vi "Main_PXI_Test.vi"() -> ()   [LabVIEW 2018]
doc: "Main VI for the controls"
uses:
  components/PMCL Dynamic Signal Analyzer/Controls/DSA excitation specs.ctl
  components/PMCL Dynamic Signal Analyzer/Controls/DSA cycle specs.ctl
  Typedefs/StateDef_Enum.ctl
  <vilib>/Utility/error.llb/DialogType.ctl
  <vilib>/Platform/TimedLoop/XDataNode/timing_clust.ctl
  <vilib>/Platform/TimedLoop/XDataNode/nitl_modes.ctl
  <vilib>/Platform/TimedLoop/XDataNode/wakeup.ctl
  <vilib>/DAQmx/read.llb/DAQmx Read (Analog 1D DBL NChan 1Samp).vi
  <vilib>/DAQmx/write.llb/DAQmx Write (Analog DBL 1Chan 1Samp).vi
  <vilib>/DAQmx/create/channels.llb/DAQmx Create Channel (AO-Voltage-Basic).vi
  <vilib>/DAQmx/create/channels.llb/DAQmx Create Channel (AI-Voltage-Basic).vi
  <vilib>/DAQmx/configure/timing.llb/DAQmx Timing (Sample Clock).vi
  <vilib>/DAQmx/create/timing.llb/DAQmx Create Timing Source (Control Loop From Task).vi
  <vilib>/DAQmx/miscellaneous.llb/DAQmx Fill In Error Info.vi
  <vilib>/Platform/TimedLoop/XDataNode/XDataNode.xnode
  Components/Timing/Timing.lvlib
  <vilib>/Platform/TimedLoop/XDataNode/XDNodeRunTimeDep.lvlib
  <vilib>/Analysis/NI_AALPro.lvlib
  <vilib>/ptbypt/NI_PtbyPt.lvlib
  <resource>/objmgr/daqmx.rc
panel:
  in  "System Stop Button":bool
  in  "Pause chart?":bool
  in  "Controller Params":enum32{"Page 1"}(tab)
  in  "Kp":dbl=1.0 min=0.0
  in  "Controller On?":bool
  out "Status":string
  in  "Ref. Gen.":enum32{"Analog In", "Manual", "Wave Gen", "DSA"}(tab)=enum."Manual"
  in  "Ref. cmd.":dbl(slide) step=1.0 scale=-10.0..10.0 scale format="%#.1f"
  in  "Signal Cluster":T1={"phase"=0.0, "amplitude"=1.0, "frequency"=1.0, "offset"=1.0, "Signal"=enum."Square"} {"offset" format="%0.2f"; "frequency" format="%0.2f"; "amplitude" format="%0.2f"; "phase" format="%0.2f"}
  in  "Frequency\nResponse":enum16{"Plant", "RR", "CL"}(ring)
  out "DSA \nRunning?":bool
  in  "Stop \nDSA":bool
  in  "Start \nDSA":bool
  in  "DSA excitation specs":T2={"Initial Freq. [Hz]"=10.0, "Final Freq. [Hz]"=999.0, "# pts. in interval"=50, "Samping Time [s]"=0.001, "Amplitude [V]"=1.0, "Offset [V]"=0.0, "Freq Units (F: rad/s, T: Hz)"=TRUE}
  in  "Cycle Specs":T3={"Cycles To \nSettle (M)"=5, "Cycles To \nCalculate (N)"=10}
  in  "Loop Timing":enum32{"Ctrl.", "Ref. gen", "UI"}(tab)
  in  "Ctrl.\nLoop Rate (Hz)":dbl=25000.0 format="%#_4p"
  out "# Finished\nLate counter":dbl
  in  "ConvLateErrToWarning?":bool=TRUE
  out "# Finished\nLate counter":dbl
  in  "Ref. Gen.\nLoop Rate (Hz)":dbl=20000.0 format="%#_4p"
  in  "UI Loop rate (Hz)":dbl=1000.0 format="%#_6p"
  in  "Display Waveforms":enum32{"Controller Signals", "DSA "}(tab)
  out "Control Effort":dbl(graph)
  out "Waveform Chart":cluster{"Double":dbl, "Numeric":dbl}(graph)
  out "Phase Bode Plot":cluster{dbl[], dbl[]}(graph)
  out "Magnitude Bode Plot":cluster{dbl[], dbl[]}(graph)
  out "DSA Signals":cluster{"Double":dbl, "Double":dbl}(graph)
  # "Connect the Reference Signal \nto C/AI 1 of the myRIO."
  # "Pinout Config.:\nPort C/AI0 : Plant output being read           by the controller.\nPort C/AI1 : Reference signal for the control loop.\nPort C/AO0 : Control effort signal to the plant."
  # "Control Loop Timing"
  # "Ref.  Gen. Loop Timing"
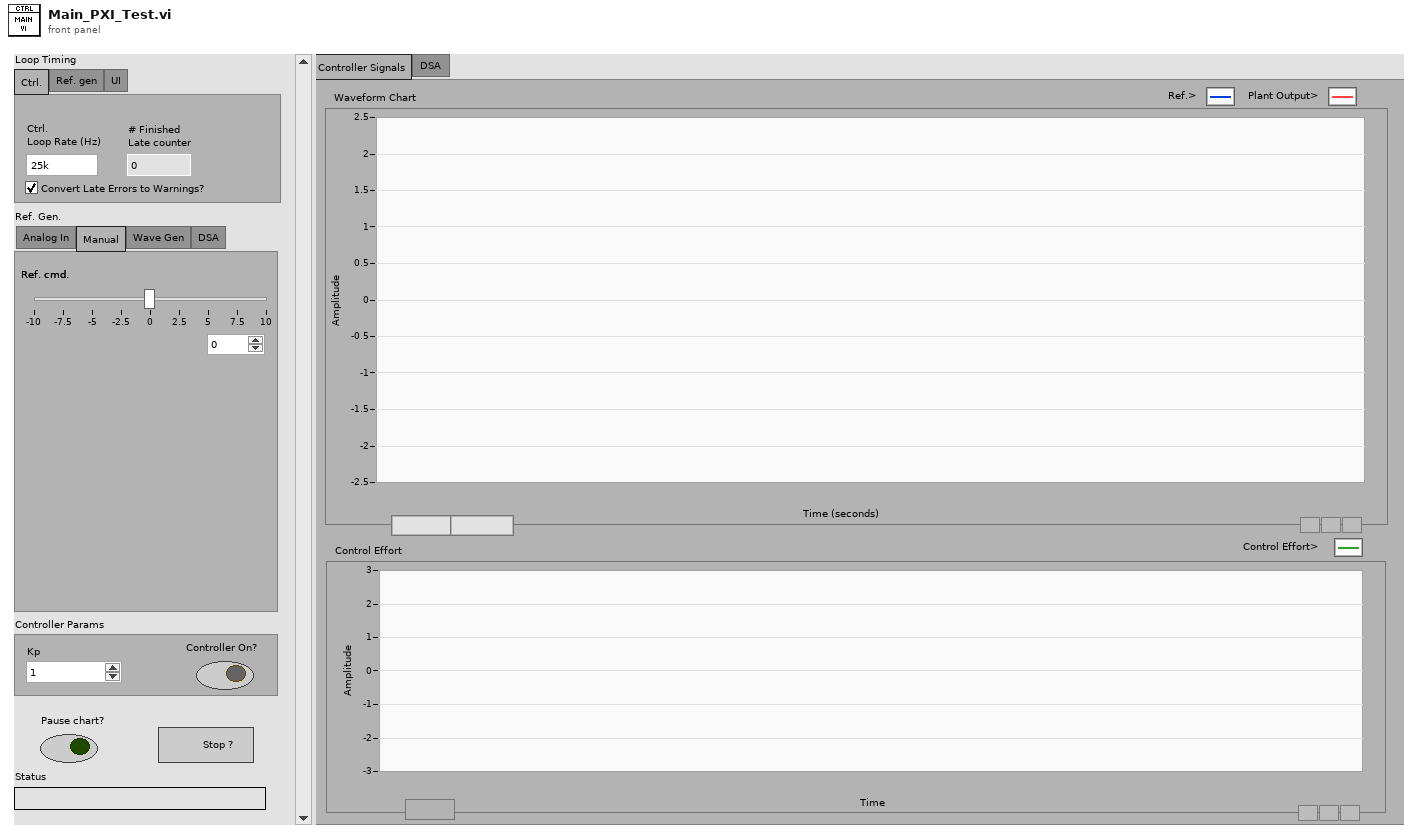
[diagram p1: front panel]
types:
  T1 = cluster{"phase":dbl, "amplitude":dbl, "frequency":dbl, "offset":dbl, "Signal":enum16{"Sine", "Square", "Sawtooth"}}
  T2 = typedef "DSA excitation specs.ctl" = cluster{"Initial Freq. [Hz]":dbl, "Final Freq. [Hz]":dbl, "# pts. in interval":i16, "Samping Time [s]":dbl, "Amplitude [V]":dbl, "Offset [V]":dbl, "Freq Units (F: rad/s, T: Hz)":bool}
  T3 = typedef "DSA cycle specs.ctl" = cluster{"Cycles To \nSettle (M)":i16, "Cycles To \nCalculate (N)":i16}
  T4 = typedef "DialogType.ctl" = u16
  T5 = typedef "StateDef_Enum.ctl" = enum16{"Initialize", "Wait", "Shutdown"}
  T6 = typedef "XDNodeRunTimeDep.lvlib/timing_clust.ctl" = cluster{"Expected End [f-1]":u64, "Actual End [f-1]":u64, "Finished Late? [f-1]":bool, "Expected End [i-1]":u64, "Actual End [i-1]":u64, "Finished Late? [i-1]":bool, "Expected Start [i]":u64, "Actual Start [i]":u64, "Expected Start [f]":u64, "Actual Start [f]":u64, "Source Name":string, "Structure Name":string, "Period":i64, "Deadline":i64, "Offset":i64, "Start":i64, "Priority":i32, "Timeout":i32, "Mode":T7, "Wakeup Reason":T8, "Error":errorcluster, "Source Type":string, "Secondary Source Type":string, "Global End Time":u64, "Global Start Time":u64, "Frame Duration":u64, "Iteration Duration":u64, "Assigned CPU":i32, "I/O Scan Engine Mode":u32}
  T7 = typedef "XDNodeRunTimeDep.lvlib/nitl_modes.ctl" = enum32{"No Change", "Process missed periods, maintain original phase", "Discard missed periods, maintain original phase", "Process missed periods, ignore original phase", "Discard missed periods, ignore original phase"}
  T8 = typedef "XDNodeRunTimeDep.lvlib/wakeup.ctl" = enum32{"Normal", "Aborted", "Asynchronous wakeup", "Timing source error", "Timed loop error", "Timeout"}
  T9 = cluster{"Analog In CH1":dbl, "Analog In CH0":dbl}
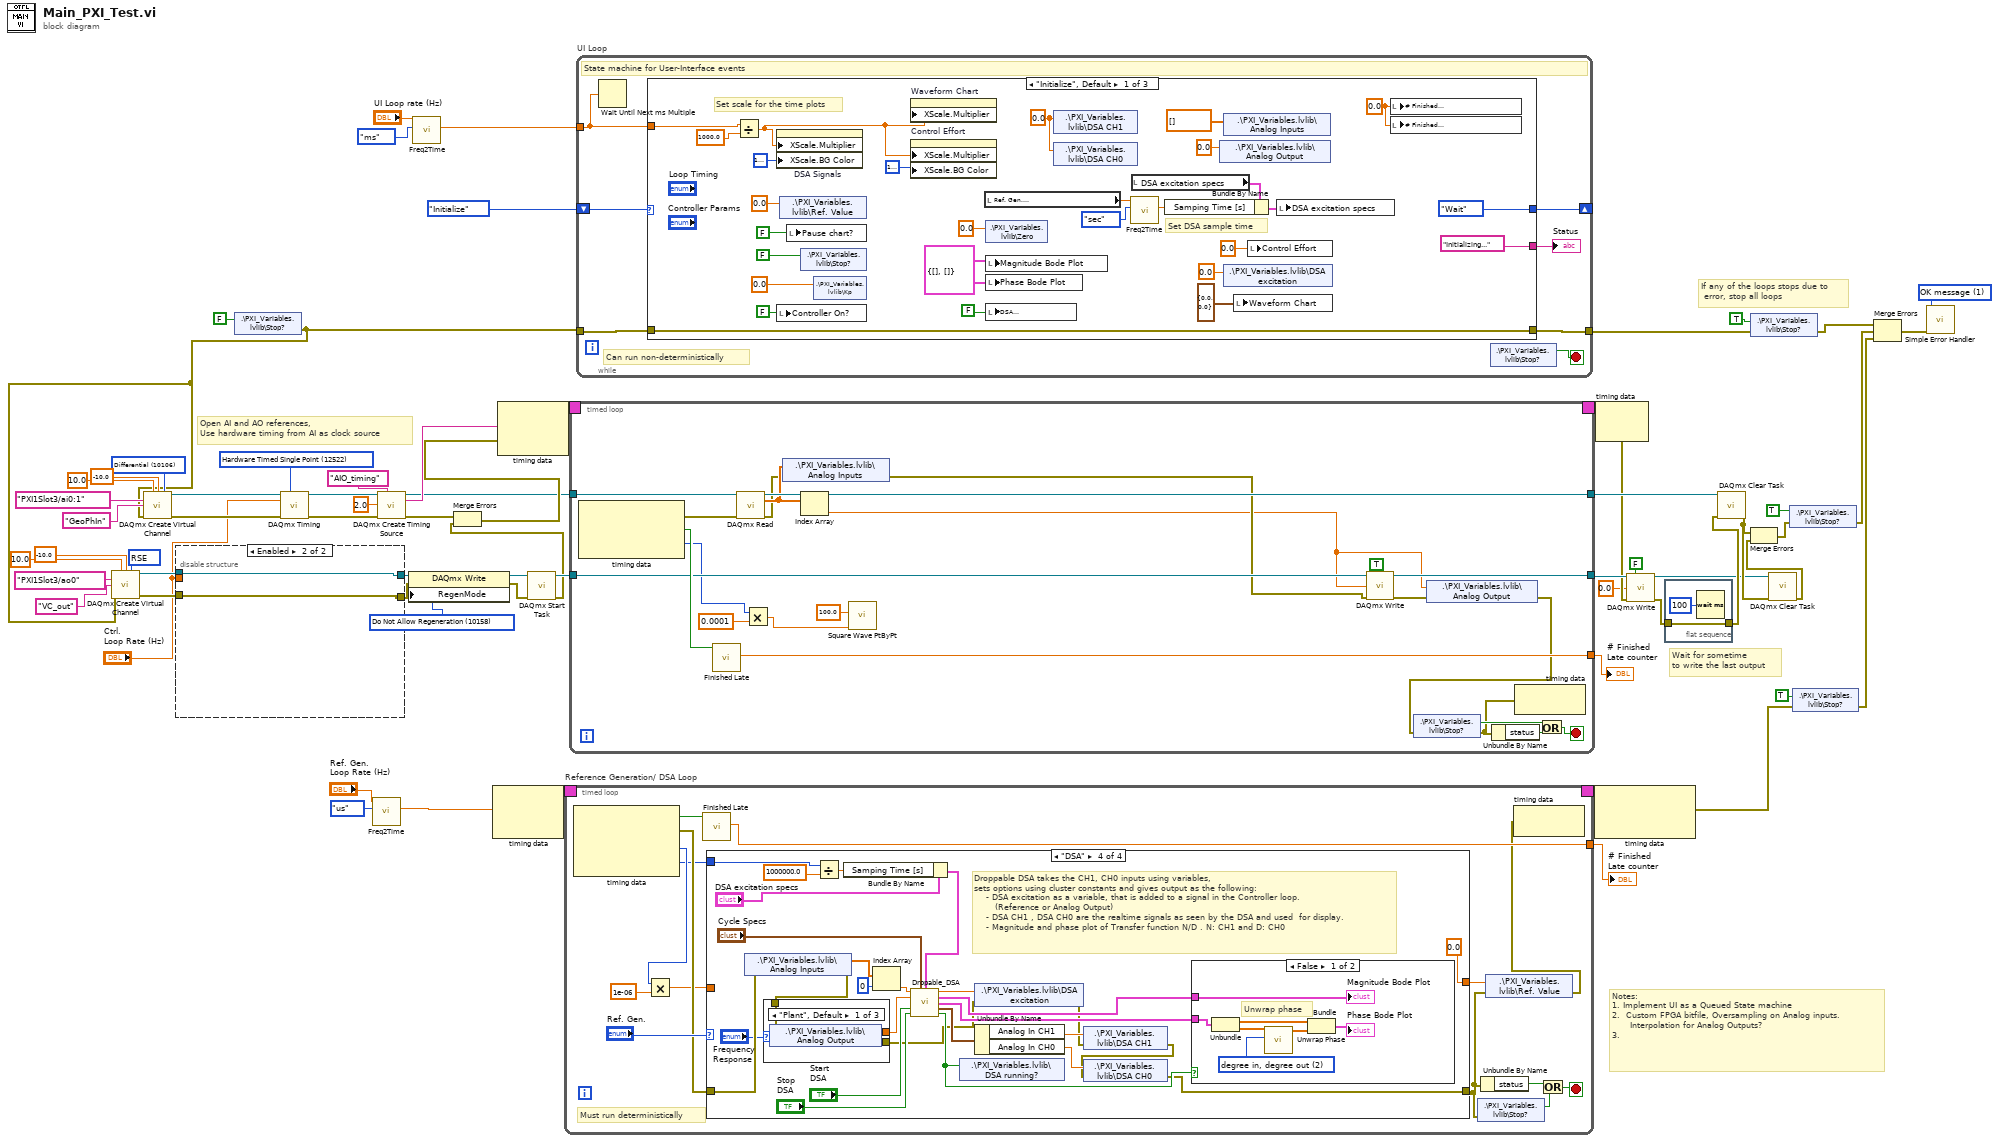
[diagram p0: block diagram]
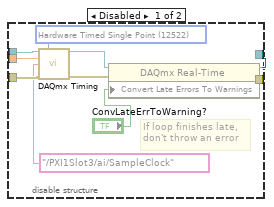
[diagram p2: hidden frame]
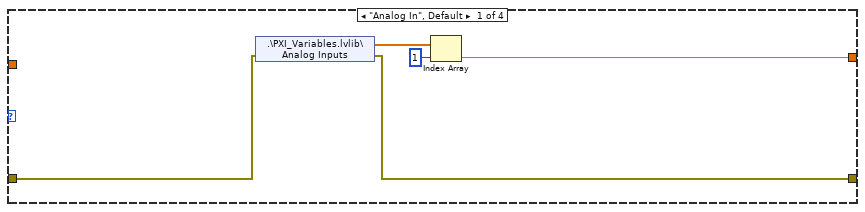
[diagram p3: hidden frame]
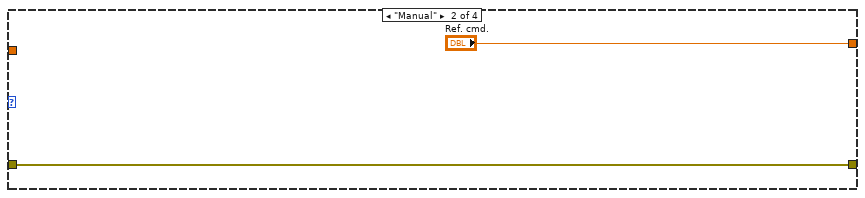
[diagram p4: hidden frame]
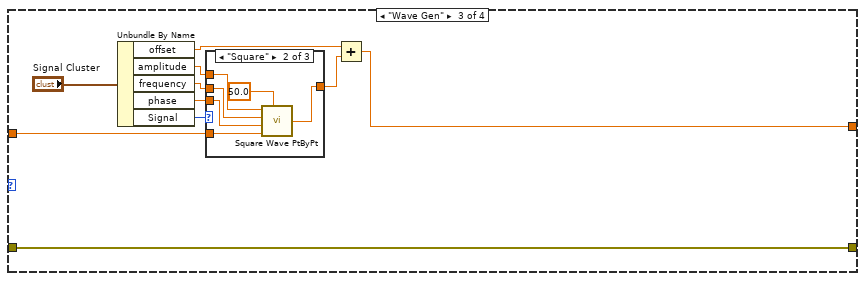
[diagram p5: hidden frame]
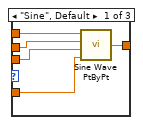
[diagram p6: hidden frame]
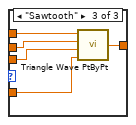
[diagram p7: hidden frame]
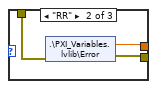
[diagram p8: hidden frame]
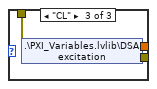
[diagram p9: hidden frame]
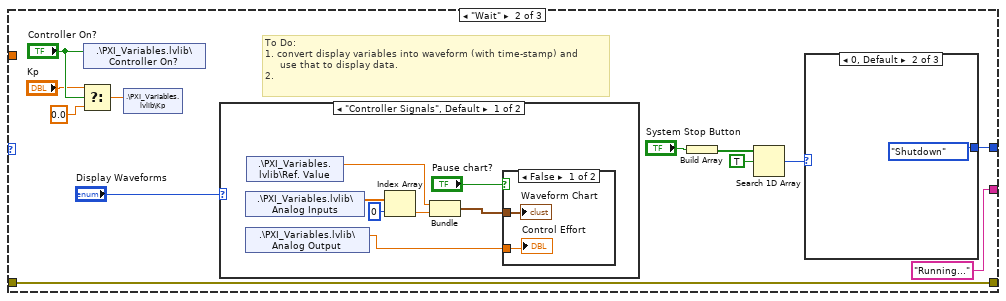
[diagram p11: hidden frame]
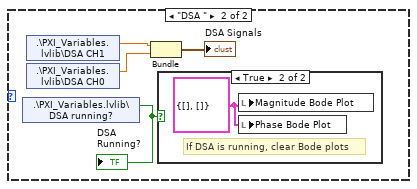
[diagram p13: hidden frame]
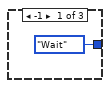
[diagram p15: hidden frame]
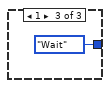
[diagram p16: hidden frame]
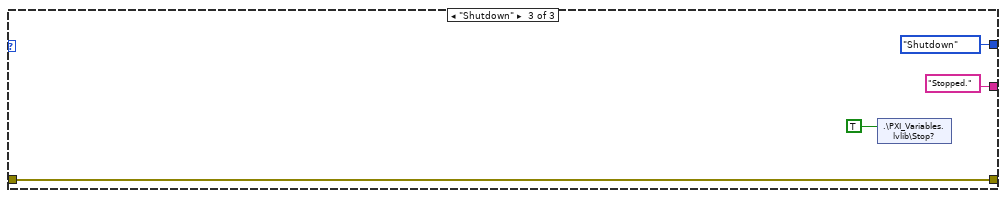
[diagram p17: hidden frame]
diagram:
  w7 = 10158 items=["Allow Regeneration"=10097, "Do Not Allow Regeneration"=10158] ("RegenMode")
  w25 = T4 1 items=["no dialog", "OK message", "continue or stop message", "OK message + warnings", "continue/stop + warnings"] ("type of dialog (OK msg:1)")
  w31 = 12522 items=["Finite Samples"=10178, "Continuous Samples"=10123, "Hardware Timed Single Point"=12522] ("sample mode")
  w47 = 10106 items=["Default"=-1, "RSE"=10083, "NRSE"=10078, "Differential"=10106, "Pseudodifferential"=12529] ("input terminal configuration")
  w50 = 10083 items=["Default"=-1, "RSE"=10083, "Differential"=10106, "Pseudodifferential"=12529] ("output terminal configuration")
  # "Wait for sometime \nto write the last output"
  # "Open AI and AO references,\nUse hardware timing from AI as clock source"
  # "Notes:\n1. Implement UI as a Queued State machine\n2.  Custom FPGA bitfile, Oversampling on Analog inputs. \n      Interpolation for Analog Outputs?\n3."
  # "If any of the loops stops due to\n error, stop all loops"
  n1 = shared-variable ".\\PXI_Variables.lvlib\\Stop?"(FALSE ("Stop?")) -> (error out=w23:errorcluster)  [unwired: 1 in]
  n2 = call-poly <vilib>:"DAQmx Create Virtual Channel.vi"("maximum value"=10.0, "minimum value"=-10.0, "output terminal configuration"=w50, "physical channels"=tag "PXI1Slot3/ao0", "name to assign"="VC_out", "error in"=w23) -> ("task out"=w11:refnum<k21>, "error out"=w10:errorcluster)  [unwired: 8 in]
  n3 = call-poly <vilib>:"DAQmx Create Virtual Channel.vi"("maximum value"=10.0, "minimum value"=-10.0, "input terminal configuration"=w47, "physical channels"=tag "PXI1Slot3/ai0:1", "name to assign"="GeoPhIn", "error in"=w23) -> ("task out"=w33:refnum<k21>, "error out"=w32:errorcluster)  [unwired: 8 in]
  n4 = disable-structure shown="Enabled" {
    disable-tunnel: w11 -> [w73 w79]
    disable-tunnel: w10 -> [w72 w78]
    disable-tunnel: "Ctrl.\nLoop Rate (Hz)" -> [w71 _]
    disable-tunnel: [w69 w78] -> w5
    disable-tunnel: [w68 w79] -> w6
    frame Disabled {
      w74 = 12522 items=["Finite Samples"=10178, "Continuous Samples"=10123, "Hardware Timed Single Point"=12522] ("sample mode")
      # "If loop finishes late,\ndon't throw an error"
      n5 = call-poly <vilib>:"DAQmx Timing.vi"("task/channels in"=w73, "sample mode"=w74, "rate"=w71, "source"=tag "/PXI1Slot3/ai/SampleClock", "error in"=w72) -> ("task out"=w76:refnum<k21>, "error out"=w75:errorcluster)  [unwired: 9 in]
      n6 = property class="DAQmx Real-Time"(reference=w76, error in=w75, "Convert Late Errors To Warnings"="ConvLateErrToWarning?") -> (reference out=w68:refnum<k21>, error out=w69:errorcluster)
    }
    frame Enabled {
    }
  }
  n7 = call-poly <vilib>:"DAQmx Timing.vi"("task/channels in"=w33, "sample mode"=w31, "rate"="Ctrl.\nLoop Rate (Hz)", "error in"=w32) -> ("task out"=w26:refnum<k21>, "error out"=w28:errorcluster)  [unwired: 10 in]
  n8 = call "Freq2Time.vi"("Int. Time Unit"=enum16{"sec", "us", "ms"}."us", "Sample rate (Hz)"="Ref. Gen.\nLoop Rate (Hz)") -> ("Int.  time [unit]"=w22:dbl)  [unwired: 7 in, 2 out]
  n9 = call-poly <vilib>:"DAQmx Create Timing Source.vi"("task/channels in"=w26, "timing source name"="AIO_timing", "sleep time (us)"=2.0, "error in"=w28) -> ("task out"=w29:refnum<k21>, "timing source out"=w30:string, "error out"=w27:errorcluster)  [unwired: 9 in]
  n10 = property class="DAQmx Write"(reference=w6, error in=w5, "RegenMode"=w7) -> (reference out=w4:refnum<k21>, error out=w2:errorcluster)
  n11 = call "Freq2Time.vi"("Int. Time Unit"=enum16{"sec", "us", "ms"}."ms", "Sample rate (Hz)"="UI Loop rate (Hz)") -> ("Int.  time [unit]"=w58:dbl)  [unwired: 7 in, 2 out]
  n12 = node-c288(w22) -> (w65:T6)  [unwired: 1 in]
  n13 = call <vilib>:"DAQmx Start Task.vi"("task/channels in"=w4, "error in"=w2) -> ("task out"=w3:refnum<k21>, "error out"=w1:errorcluster)  [unwired: 12 in]
  n14 = Merge Errors(w27, w1) -> (w41:errorcluster)
  n15 = node-c288(w30, w41) -> (w43:T6)
  n16 = timed-loop "Reference Generation/ DSA Loop" {
    timing: w65 -> [_]
    timing-out: [_] -> w64
    tunnel: [w92] -> w63
    stop <- w86 stop-if-true
    # "Must run deterministically"
    n17 = node-c288() -> (w93:bool, w89:errorcluster, w83:i64, w82:i64)  [unwired: 1 in]
    n18 = Multiply(x=w83, y=1e-06) -> (x*y=w85:dbl)
    n19 = call "Finished Late.vi"("Finished \nLate?"=w93) -> ("# Finished\nLate counter"=w92:dbl)  [unwired: 8 in, 2 out]
    n20 = case shown="\"DSA\"" "Ref. Gen." {
      tunnel: [w98 "Ref. cmd." w103 0.0 ("Ref. cmd.")] -> w90
      tunnel: w89 -> [w96 w99 w102 w133]
      tunnel: [w95 w99 w102 w136] -> w80
      tunnel: w85 -> [_ _ w101 _]
      tunnel: w82 -> [_ _ _ w143]
      frame "Analog In", Default {
        n21 = shared-variable ".\\PXI_Variables.lvlib\\Analog Inputs"(error in=w96) -> (w97:dbl[], error out=w95:errorcluster)
        n22 = Index Array(array=w97, index=1) -> (element=w98:dbl)
      }
      frame "Manual" {
      }
      frame "Wave Gen" {
        n23 = Unbundle By Name("Signal Cluster") -> ("offset"=w104:dbl, "amplitude"=w107:dbl, "frequency"=w106:dbl, "phase"=w105:dbl, "Signal"=w108:enum16{"Sine", "Square", "Sawtooth"})
        n24 = case shown="\"Square\"" w108 {
          tunnel: [w115 w120 w126] -> w110
          tunnel: w107 -> [w114 w119 w125]
          tunnel: w106 -> [w113 w118 w124]
          tunnel: w105 -> [w112 w117 w123]
          tunnel: w101 -> [w111 w116 w122]
          frame "Sine", Default {
            n25 = call <vilib>:"Sine Wave PtByPt.vi"("time"=w111, "phase"=w112, "frequency"=w113, "amplitude"=w114) -> ("sine wave"=w115:dbl)
          }
          frame "Square" {
            n26 = call <vilib>:"Square Wave PtByPt.vi"("amplitude"=w119, "frequency"=w118, "phase"=w117, "time"=w116, "duty cycle (%)"=50.0) -> ("square wave"=w120:dbl)
          }
          frame "Sawtooth" {
            n27 = call <vilib>:"Triangle Wave PtByPt.vi"("time"=w122, "phase"=w123, "frequency"=w124, "amplitude"=w125) -> ("triangle wave"=w126:dbl)
          }
        }
        n28 = Add(x=w104, y=w110) -> (x+y=w103:dbl)
      }
      frame "DSA" {
        # "Droppable DSA takes the CH1, CH0 inputs using variables, \nsets options using cluster constants and gives output as the following:\n    - DSA excitation as a variable, that is added to a signal in the Controller loop. \n       (Reference or Analog Output)\n    - DSA CH1 , DSA CH0 are the realtime signals as seen by the DSA and used  for display.\n    - Magnitude and phase plot of Transfer function N/D . N: CH1 and D: CH0"
        n29 = shared-variable ".\\PXI_Variables.lvlib\\Analog Inputs"(error in=w133) -> (w132:dbl[], error out=w130:errorcluster)
        n30 = case shown="\"Plant\", Default" "Frequency\nResponse" {
          tunnel: [w156 w159 w160] -> w131
          tunnel: w130 -> [w155 w157 w162]
          tunnel: [w154 w158 w161] -> w127
          frame "Plant", Default {
            n31 = shared-variable ".\\PXI_Variables.lvlib\\Analog Output"(error in=w155) -> (w156:dbl, error out=w154:errorcluster)
          }
          frame "RR" {
            n32 = shared-variable ".\\PXI_Variables.lvlib\\Error"(error in=w157) -> (w159:dbl, error out=w158:errorcluster)
          }
          frame "CL" {
            n33 = shared-variable ".\\PXI_Variables.lvlib\\DSA excitation"(error in=w162) -> (w160:dbl, error out=w161:errorcluster)
          }
        }
        n34 = Divide(x=w143, y=1000000.0) -> (x/y=w141:dbl)
        n35 = Bundle By Name(cluster="DSA excitation specs", "Samping Time [s]"=w141) -> (w140:T2)
        n36 = Index Array(array=w132, index=0) -> (element=w134:dbl)
        n37 = call "Dropable_DSA.vi"("Analog In CH1"=w134, "Cycle Specs"="Cycle Specs", "Excitation Specs"=w140, "Analog In CH0"=w131, "START"="Start \nDSA", "STOP"="Stop \nDSA") -> ("Analog Out"=w152:dbl, "Bode Magnitude"=w145:cluster{dbl[], dbl[]}, "Bode Phase"=w144:cluster{dbl[], dbl[]}, "Live signals"=w149:T9, "Running"=w139:bool)  [unwired: 4 in, 1 out]
        n38 = shared-variable ".\\PXI_Variables.lvlib\\DSA running?"(w139) -> ()  [unwired: 1 in, 1 out]
        n39 = shared-variable ".\\PXI_Variables.lvlib\\DSA excitation"(w152, error in=w127) -> (error out=w138:errorcluster)
        n40 = Unbundle By Name(w149) -> ("Analog In CH1"=w148:dbl, "Analog In CH0"=w147:dbl)
        n41 = shared-variable ".\\PXI_Variables.lvlib\\DSA CH1"(w148, error in=w138) -> (error out=w137:errorcluster)
        n42 = shared-variable ".\\PXI_Variables.lvlib\\DSA CH0"(w147, error in=w137) -> (error out=w136:errorcluster)
        n43 = case shown="False" w139 {
          tunnel: w145 -> [w163 _]
          tunnel: w144 -> [w165 _]
          frame False {
            w167 = 2 items=["radian in, radian out", "radian in, degree out", "degree in, degree out", "degree in, radian out"] ("phase unit")
            # "Unwrap phase"
            n44 = Unbundle(w165) -> (w169:dbl[], w166:dbl[])
            n45 = call <vilib>:"Unwrap Phase.vi"("phase unit"=w167, "Phase"=w166) -> ("Unwrapped Phase"=w168:dbl[])  [unwired: 8 in, 1 out]
            n46 = Bundle(w169, "Unwrapped Phase"=w168) -> (→"Phase Bode Plot":cluster{dbl[], "Unwrapped Phase":dbl[]})  [unwired: 1 in]
            "Magnitude Bode Plot" <- w163
          }
          frame True {
          }
        }
      }
    }
    n47 = shared-variable ".\\PXI_Variables.lvlib\\Stop?"(error in=w80) -> (w87:bool)  [unwired: 1 out]
    n48 = Unbundle By Name(w80) -> ("status"=w88:bool)
    n49 = shared-variable ".\\PXI_Variables.lvlib\\Ref. Value"(w90, error in=w80) -> (error out=w81:errorcluster)
    n50 = node-c288(w81) -> ()  [unwired: 1 out]
    n51 = Or(x=w88, y=w87) -> (x .or. y?=w86:bool)
  }
  "# Finished\nLate counter" <- w63
  n52 = timed-loop {
    timing: w43 -> [_]
    timing-out: [_] -> w42
    tunnel: w29 -> [w198]
    tunnel: [w196] -> w35
    tunnel: [w195] -> w34
    tunnel: w3 -> [w184]
    tunnel: [w189] -> w17
    stop <- w190 stop-if-true
    n53 = node-c288() -> (w199:errorcluster, w197:bool, w181:i64)  [unwired: 1 in]
    n54 = call "Finished Late.vi"("Finished \nLate?"=w197) -> ("# Finished\nLate counter"=w196:dbl)  [unwired: 8 in, 2 out]
    n55 = call-poly <vilib>:"DAQmx Read.vi"("task/channels in"=w198, "error in"=w199) -> ("task out"=w195:refnum<k21>, "data"=w194:dbl[], "error out"=w188:errorcluster)  [unwired: 11 in]
    n56 = Multiply(x=w181, y=0.0001) -> (x*y=w180:dbl)
    n57 = shared-variable ".\\PXI_Variables.lvlib\\Analog Inputs"(w194, error in=w188) -> (error out=w183:errorcluster)
    n58 = Index Array(array=w194) -> (element=w178:dbl)  [unwired: 1 in]
    n59 = call <vilib>:"Square Wave PtByPt.vi"("frequency"=100.0, "time"=w180) -> ()  [unwired: 3 in, 1 out]
    n60 = call-poly <vilib>:"DAQmx Write.vi"("task/channels in"=w184, "auto start"=TRUE, "data"=w178, "error in"=w183) -> ("task out"=w189:refnum<k21>, "error out"=w187:errorcluster)  [unwired: 9 in, 1 out]
    n61 = shared-variable ".\\PXI_Variables.lvlib\\Analog Output"(w178, error in=w187) -> (error out=w186:errorcluster)
    n62 = shared-variable ".\\PXI_Variables.lvlib\\Stop?"(error in=w186) -> (w193:bool, error out=w192:errorcluster)
    n63 = Unbundle By Name(w192) -> ("status"=w191:bool)
    n64 = node-c288(w192) -> ()  [unwired: 1 out]
    n65 = Or(x=w193, y=w191) -> (x .or. y?=w190:bool)
  }
  "# Finished\nLate counter" <- w35
  n66 = while "UI Loop" {
    shift-right: [w212] -> _
    shift-left: StateDef_Enum."Initialize" ("State defining Enum") -> [w213]
    tunnel: w23 -> [w211]
    tunnel: [w210] -> w57
    tunnel: w58 -> [w207]
    stop <- w208 stop-if-true
    # "Can run non-deterministically"
    # "State machine for User-Interface events"
    n67 = Wait Until Next ms Multiple(millisecond multiple=w207) -> ()  [unwired: 1 out]
    n68 = case shown="\"Initialize\", Default" w213 {
      tunnel: [StateDef_Enum."Wait" ("State defining Enum") w250 StateDef_Enum."Shutdown" ("State defining Enum")] -> w212
      tunnel: w211 -> [w238 w248 w274]
      tunnel: [w238 w248 w274] -> w210
      tunnel: ["Initializing..." ("Status") "Running..." ("Status") "Stopped." ("Status")] -> w209
      tunnel: w207 -> [w236 _ _]
      frame "Initialize", Default {
        w214 = 0.0 ("# Finished\nLate counter")
        w215 = 0.0 ("DSA CH1")
        w231 = cluster{dbl[], dbl[]} {[], []} ("Magnitude Bode Plot")
        # "Set DSA sample time"
        # "Set scale for the time plots"
        n69 = Divide(x=w236, y=1000.0) -> (x/y=w223:dbl)
        n70 = property on="DSA Signals" class="WFChart (strict)"("XScale.Multiplier"=w223, "XScale.BG Color"=u32 16777216) -> ()  [unwired: 2 in, 2 out]
        n71 = local write "Controller On?"(FALSE ("Controller On?")) -> ()
        n72 = shared-variable ".\\PXI_Variables.lvlib\\Ref. Value"(0.0 ("Ref. Value")) -> ()  [unwired: 1 in, 1 out]
        n73 = local write "Pause chart?"(FALSE ("Pause chart?")) -> ()
        n74 = shared-variable ".\\PXI_Variables.lvlib\\Stop?"(FALSE ("Stop?")) -> ()  [unwired: 1 in, 1 out]
        n75 = shared-variable ".\\PXI_Variables.lvlib\\Kp"(0.0 ("Kp")) -> ()  [unwired: 1 in, 1 out]
        n76 = property on="Waveform Chart" class="WFChart (strict)"("XScale.Multiplier"=w223) -> ()  [unwired: 2 in, 2 out]
        n77 = property on="Control Effort" class="WFChart (strict)"("XScale.Multiplier"=w223, "XScale.BG Color"=u32 16777216) -> ()  [unwired: 2 in, 2 out]
        n78 = local read "Ref. Gen.\nLoop Rate (Hz)"() -> (w226:dbl)
        n79 = shared-variable ".\\PXI_Variables.lvlib\\Zero"(0.0 ("Zero")) -> ()  [unwired: 1 in, 1 out]
        n80 = local write "Magnitude Bode Plot"(w231) -> ()
        n81 = local write "Phase Bode Plot"(w231) -> ()
        n82 = local write "DSA \nRunning?"(FALSE ("DSA \nRunning?")) -> ()
        n83 = shared-variable ".\\PXI_Variables.lvlib\\DSA CH1"(w215) -> ()  [unwired: 1 in, 1 out]
        n84 = shared-variable ".\\PXI_Variables.lvlib\\DSA CH0"(w215) -> ()  [unwired: 1 in, 1 out]
        n85 = call "Freq2Time.vi"("Int. Time Unit"=enum16{"sec", "us", "ms"}."sec", "Sample rate (Hz)"=w226) -> ("Int.  time [unit]"=w224:dbl)  [unwired: 7 in, 2 out]
        n86 = local read "DSA excitation specs"() -> (w228:T2)
        n87 = Bundle By Name(cluster=w228, "Samping Time [s]"=w224) -> (w227:T2)
        n88 = shared-variable ".\\PXI_Variables.lvlib\\Analog Output"(0.0 ("Analog Output")) -> ()  [unwired: 1 in, 1 out]
        n89 = shared-variable ".\\PXI_Variables.lvlib\\Analog Inputs"(dbl[] [] ("Analog Inputs")) -> ()  [unwired: 1 in, 1 out]
        n90 = shared-variable ".\\PXI_Variables.lvlib\\DSA excitation"(0.0 ("DSA excitation")) -> ()  [unwired: 1 in, 1 out]
        n91 = local write "Waveform Chart"(cluster{"Double":dbl, "Numeric":dbl} {"Double"=0.0, "Numeric"=0.0} ("Waveform Chart")) -> ()
        n92 = local write "Control Effort"(0.0 ("Control Effort")) -> ()
        n93 = local write "DSA excitation specs"(w227) -> ()
        n94 = local write "# Finished\nLate counter"(w214) -> ()
        n95 = local write "# Finished\nLate counter"(w214) -> ()
      }
      frame "Wait" {
        # "To Do:\n1. convert display variables into waveform (with time-stamp) and\n     use that to display data.\n2."
        n96 = Select(t="Kp", s="Controller On?", f=0.0) -> (s? t:f=w246:dbl)
        n97 = shared-variable ".\\PXI_Variables.lvlib\\Controller On?"("Controller On?") -> ()  [unwired: 1 in, 1 out]
        n98 = shared-variable ".\\PXI_Variables.lvlib\\Kp"(w246) -> ()  [unwired: 1 in, 1 out]
        n99 = case shown="\"Controller Signals\", Default" "Display Waveforms" {
          frame "Controller Signals", Default {
            n100 = shared-variable ".\\PXI_Variables.lvlib\\Analog Inputs"() -> (w260:dbl[])  [unwired: 1 in, 1 out]
            n101 = shared-variable ".\\PXI_Variables.lvlib\\Analog Output"() -> (w254:dbl)  [unwired: 1 in, 1 out]
            n102 = shared-variable ".\\PXI_Variables.lvlib\\Ref. Value"() -> (w257:dbl)  [unwired: 1 in, 1 out]
            n103 = Index Array(array=w260, index=0) -> (element=w259:dbl)
            n104 = Bundle("Double"=w257, "Numeric"=w259) -> (w255:cluster{"Double":dbl, "Numeric":dbl})  [unwired: 1 in]
            n105 = case shown="False" "Pause chart?" {
              tunnel: w255 -> [w262 _]
              tunnel: w254 -> [w261 _]
              frame False {
                "Waveform Chart" <- w262
                "Control Effort" <- w261
              }
              frame True {
              }
            }
          }
          frame "DSA " {
            n106 = shared-variable ".\\PXI_Variables.lvlib\\DSA running?"() -> (w263:bool)  [unwired: 1 in, 1 out]
            "DSA \nRunning?" <- w263
            n107 = shared-variable ".\\PXI_Variables.lvlib\\DSA CH1"() -> (w265:dbl)  [unwired: 1 in, 1 out]
            n108 = shared-variable ".\\PXI_Variables.lvlib\\DSA CH0"() -> (w264:dbl)  [unwired: 1 in, 1 out]
            n109 = Bundle("Double"=w265, "Double"=w264) -> (→"DSA Signals":cluster{"Double":dbl, "Double":dbl})  [unwired: 1 in]
            n110 = case shown="True" w263 {
              frame False {
              }
              frame True {
                w267 = cluster{dbl[], dbl[]} {[], []} ("Magnitude Bode Plot")
                # "If DSA is running, clear Bode plots"
                n111 = local write "Magnitude Bode Plot"(w267) -> ()
                n112 = local write "Phase Bode Plot"(w267) -> ()
              }
            }
          }
        }
        n113 = Build Array("System Stop Button") -> (w252:bool[])
        n114 = Search 1D Array(1D array=w252, element=TRUE) -> (index of element=w249:i32)  [unwired: 1 in]
        n115 = case shown="0, Default" w249 {
          tunnel: [StateDef_Enum."Wait" ("State defining Enum") StateDef_Enum."Shutdown" ("State defining Enum") StateDef_Enum."Wait" ("State defining Enum")] -> w250
          frame -1 {
          }
          frame 0, Default {
          }
          frame 1 {
          }
        }
      }
      frame "Shutdown" {
        n116 = shared-variable ".\\PXI_Variables.lvlib\\Stop?"(TRUE) -> ()  [unwired: 1 in, 1 out]
      }
    }
    "Status" <- w209
    n117 = shared-variable ".\\PXI_Variables.lvlib\\Stop?"() -> (w208:bool)  [unwired: 1 in, 1 out]
  }
  n118 = node-c288(w64) -> (w62:errorcluster)  [unwired: 1 out]
  n119 = node-c288(w42) -> (w16:errorcluster)
  n120 = call-poly <vilib>:"DAQmx Write.vi"("task/channels in"=w17, "auto start"=FALSE, "data"=0.0, "error in"=w16) -> ("task out"=w12:refnum<k21>, "error out"=w14:errorcluster)  [unwired: 9 in, 1 out]
  n121 = flat-sequence {
    tunnel: [w276] -> w13
    tunnel: w14 -> [w276]
    frame #0 {
      n122 = Wait (ms)(milliseconds to wait=u32 100) -> ()  [unwired: 1 out]
    }
  }
  n123 = call <vilib>:"DAQmx Clear Task.vi"("task in"=w34, "error in"=w13) -> ("error out"=w18:errorcluster)  [unwired: 13 in]
  n124 = shared-variable ".\\PXI_Variables.lvlib\\Stop?"(TRUE ("Stop?"), error in=w57) -> (error out=w56:errorcluster)
  n125 = call <vilib>:"DAQmx Clear Task.vi"("task in"=w12, "error in"=w18) -> ("error out"=w38:errorcluster)  [unwired: 13 in]
  n126 = Merge Errors(w18, w38) -> (w39:errorcluster)
  n127 = shared-variable ".\\PXI_Variables.lvlib\\Stop?"(TRUE ("Stop?"), error in=w39) -> (error out=w36:errorcluster)
  n128 = shared-variable ".\\PXI_Variables.lvlib\\Stop?"(TRUE ("Stop?"), error in=w62) -> (error out=w37:errorcluster)
  n129 = Merge Errors(w56, w36, w37) -> (w66:errorcluster)
  n130 = call <vilib>:"Simple Error Handler.vi"("type of dialog (OK msg:1)"=w25, "error in (no error)"=w66) -> ()  [unwired: 3 in, 5 out]
